vi "Reserve.vi"(8 "error in (no error)":errorcluster, 10 "Purpose":string, 11 "Resource in":refnum<class "Resource.lvclass">) -> (0 "error out":errorcluster, 3 "Resource out":refnum<class "Resource.lvclass">)   [LabVIEW 2020, in "CTI.lvlib" / "Resource.lvclass"]
uses:
  Resource.lvclass
  Resource.lvclass/Resource.ctl
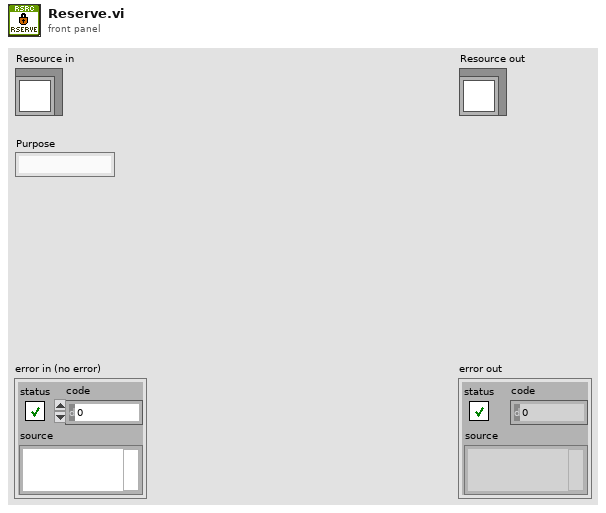
[diagram p1: front panel]
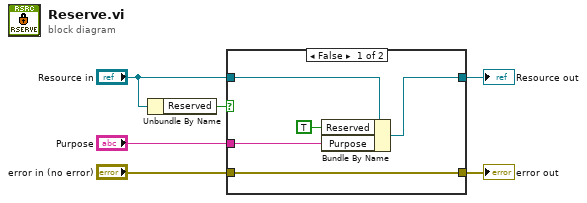
[diagram p0: block diagram]
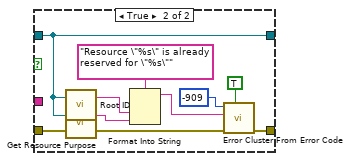
[diagram p2: hidden frame]
diagram:
  n1 = Unbundle By Name("Resource in") -> ("Reserved"=w1:bool)
  n2 = case shown="False" w1 {
    tunnel: [w11 w16] -> w6
    tunnel: "Purpose" -> [w9 _]
    tunnel: "Resource in" -> [w8 w16]
    tunnel: "error in (no error)" -> [w7 w20]
    tunnel: [w7 w19] -> w2
    frame False {
      n3 = Bundle By Name(cluster=w8, "Reserved"=TRUE, "Purpose"=w9) -> (w11:refnum<class "Resource.lvclass">)
    }
    frame True {
      n4 = call "Root ID.vi"("Resource in"=w16) -> ("Root ID"=w15:string)  [unwired: 6 in]
      n5 = call "Get Resource Purpose.vi"("Resource in"=w16) -> ("Resource Purpose"=w14:string)  [unwired: 6 in]
      n6 = Format Into String(format string="Resource \"%s\" is already reserved for \"%s\"", w15, w14) -> (resulting string=w13:string)  [unwired: 2 in, 1 out]
      n7 = call <vilib>:"Error Cluster From Error Code.vi"("show call chain? (False)"=TRUE, "error in (no error)"=w20, "error message (\"\")"=w13, "error code (0)"=-909) -> ("error out"=w19:errorcluster)  [unwired: 5 in]
    }
  }
  "error out" <- w2
  "Resource out" <- w6
